vi "Compensation.vi"(5 "Impedance Comp Mode(F:Interpolation)":bool, 6 "Gain-Phase DataB Offset(T:On)":bool=TRUE, 7 "ImpedancePhaseScale(F:Normal)":bool, 8 "error in (no error)":errorcluster, 9 "Gain-Phase DataA Offset(F:Off)":bool, 10 "Store Offset Reference (T:On)":bool=TRUE, 11 "VISA resource name":refnum<visa-resource-name>) -> (0 "error out":errorcluster, 3 "VISA resource name out":refnum<visa-resource-name>)   [LabVIEW 2010, in "Agilent 4194.lvlib"]
doc: "This function sets the compensation parameters for impedance and phase-gain modes."
uses:
  <instrlib>/Agilent 4194/Agilent 4194.lvlib
panel:
  # "All Points\nInterpolation"
  # "Expansion\nNormal"
  # "On\nOff"
  # "On\nOff"
  # "On\nOff"
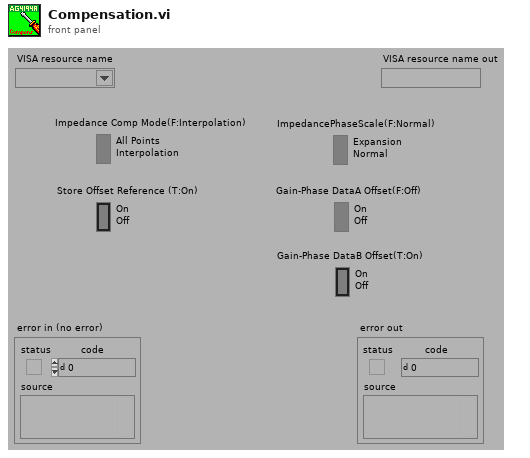
[diagram p1: front panel]
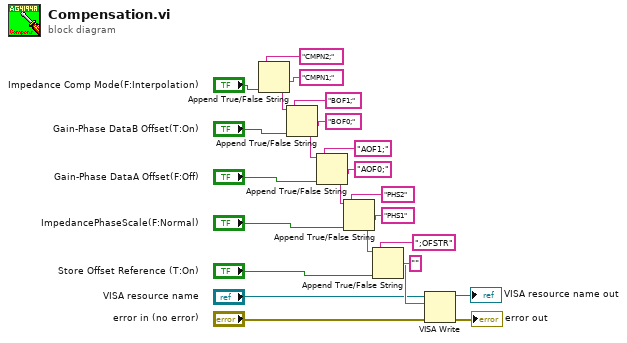
[diagram p0: block diagram]
diagram:
  n1 = Append True/False String(1:"Impedance Comp Mode(F:Interpolation)", 2:"CMPN1;", 3:"CMPN2;") -> (0:w14:string)  [unwired: 1 in]
  n2 = Append True/False String(1:"Gain-Phase DataB Offset(T:On)", 2:"BOF0;", 3:"BOF1;", 4:w14) -> (0:w13:string)
  n3 = Append True/False String(1:"Gain-Phase DataA Offset(F:Off)", 2:"AOF0;", 3:"AOF1;", 4:w13) -> (0:w12:string)
  n4 = Append True/False String(1:"ImpedancePhaseScale(F:Normal)", 2:"PHS1", 3:"PHS2", 4:w12) -> (0:w11:string)
  n5 = Append True/False String(1:"Store Offset Reference (T:On)", 2:"", 3:";OFSTR", 4:w11) -> (0:w10:string)
  n6 = VISA Write(VISA resource name="VISA resource name", write buffer=w10, error in (no error)="error in (no error)") -> (VISA resource name out=→"VISA resource name out":refnum<visa-resource-name>, error out=→"error out":errorcluster)  [unwired: 1 out]
